vi "Process.vi"(0 "reference in":refnum<class "Active object Event.lvclass">, 5 "error in (no error)":errorcluster) -> (14 "reference out":refnum<class "Active object Event.lvclass">, 19 "error out":errorcluster)   [LabVIEW 2019, in "Active object Event.lvclass"]
uses:
  Active object Event.lvclass
panel:
  out "Last Command":string
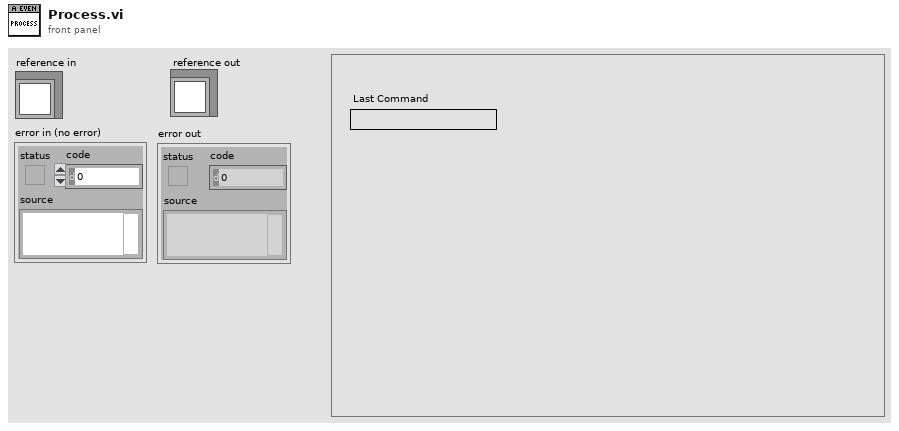
[diagram p1: front panel]
types:
  T1 = cluster{"Event":refnum<event-registration>, "Command":string, "Data":variant}
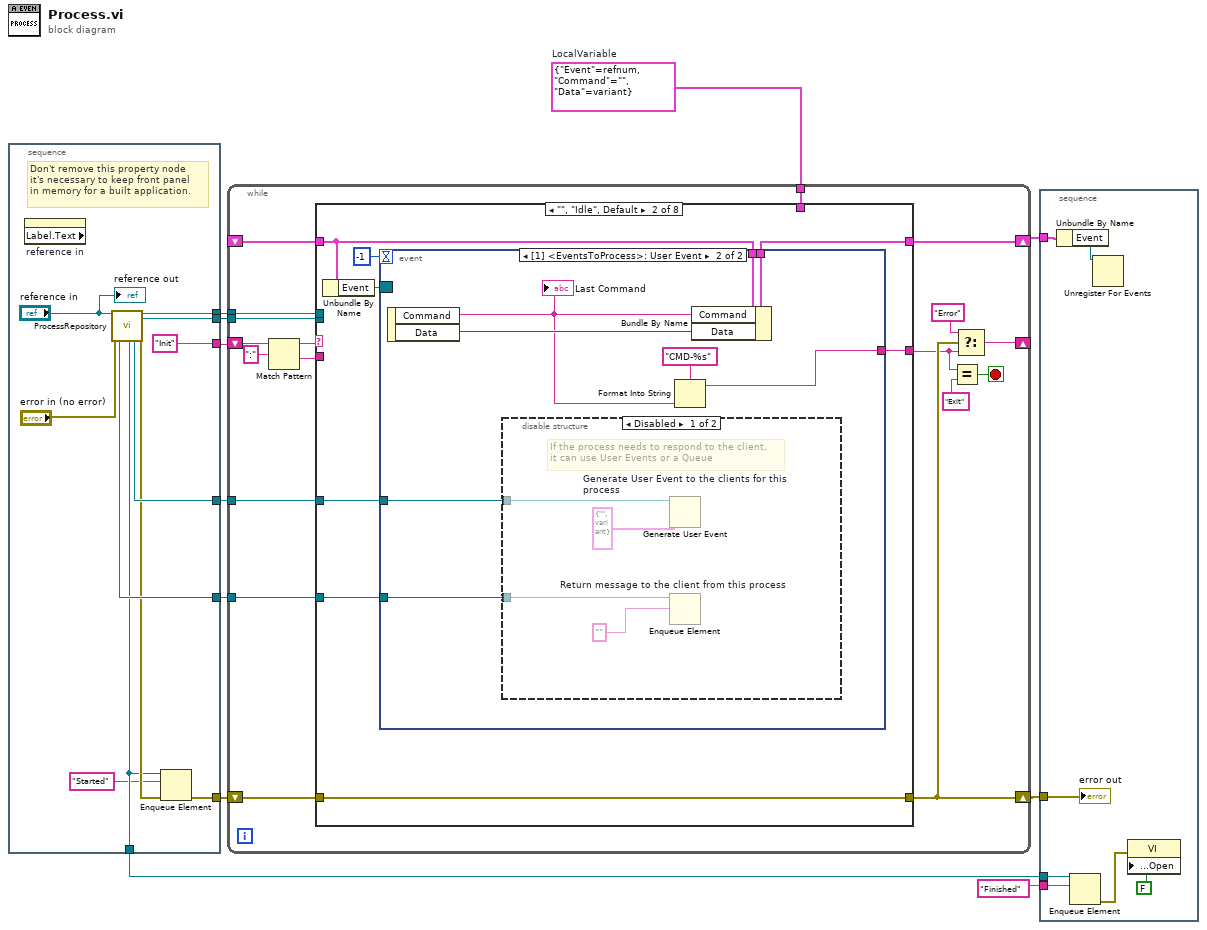
[diagram p0: block diagram]
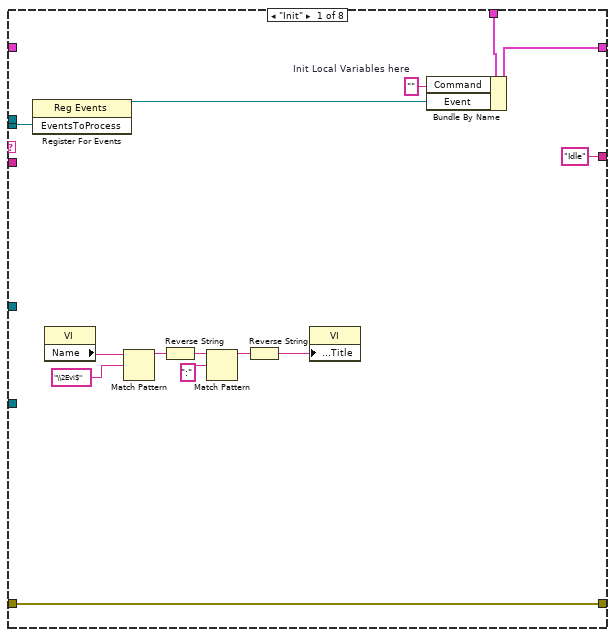
[diagram p2: hidden frame]
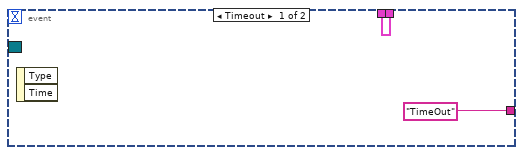
[diagram p3: hidden frame]
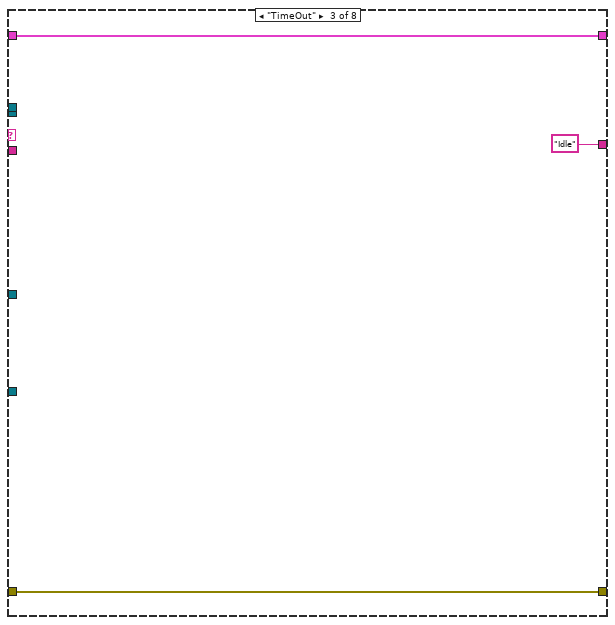
[diagram p5: hidden frame]
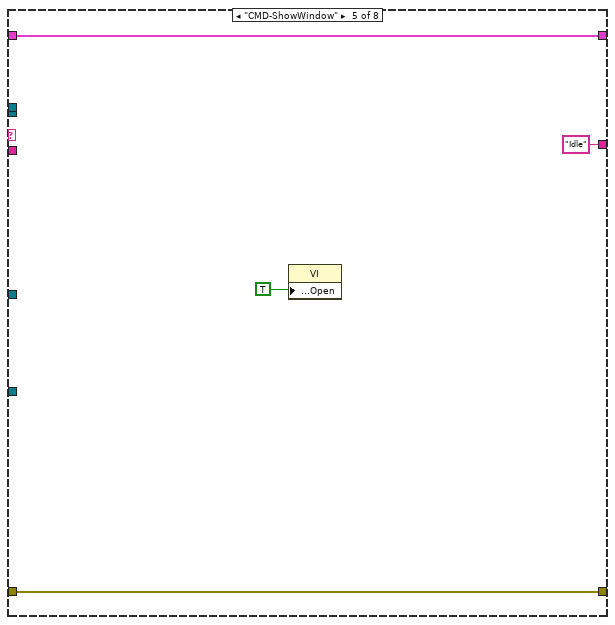
[diagram p7: hidden frame]
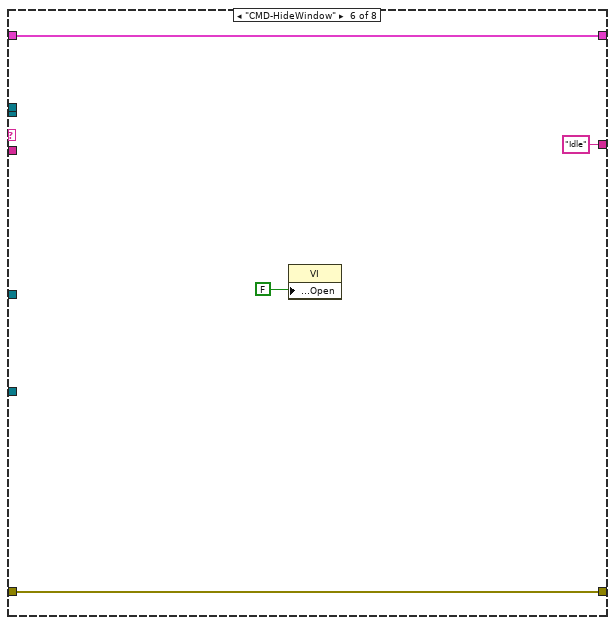
[diagram p8: hidden frame]
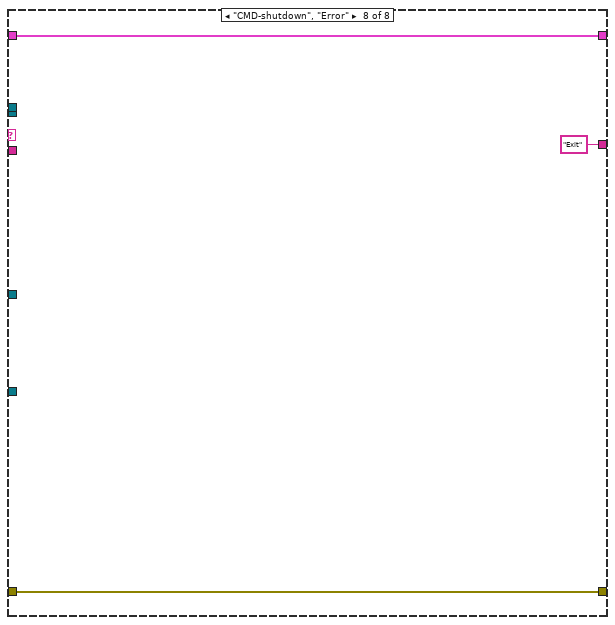
[diagram p10: hidden frame]
diagram:
  w5 = T1 {"Event"=refnum, "Command"="", "Data"=variant}  # LocalVariable
  n1 = stacked-sequence {
    tunnel: [w13] -> w11
    tunnel: [w22] -> w9
    tunnel: [w19] -> w8
    tunnel: [w14] -> w7
    tunnel: ["Init"] -> w6
    tunnel: [w17] -> w3
    tunnel: [w16] -> w2
    frame #0 {
      # "Don't remove this property node\nit's necessary to keep front panel\nin memory for a built application."
      n2 = property on="reference in" class="LVClassControl (strict)" props=["Label", "Text"]() -> ()  [unwired: 2 in, 3 out]
      n3 = call "ProcessRepository.vi"("reference in"="reference in", "error in (no error)"="error in (no error)") -> ("QueueFromProcess"=w16:refnum<queue>, "ProcessSyncQueue"=w14:refnum<queue>, "EventFromProcess"=w17:refnum<user-event>, "reference out"=w22:refnum<class "Active object Event.lvclass">, "EventsToProcess"=w19:refnum<user-event>, "error out"=w15:errorcluster)  [unwired: 10 in, 2 out]
      n4 = Enqueue Element(queue=w14, element="Started", error in (no error)=w15) -> (error out=w13:errorcluster)  [unwired: 1 in, 2 out]
      "reference out" <- "reference in"
    }
  }
  n5 = while {
    shift-right: [w33] -> w10
    shift-left: w11 -> [w38]
    tunnel: w9 -> [w39]
    tunnel: w8 -> [w40]
    shift-right: [w31] -> _
    shift-left: w6 -> [w36]
    shift-right: [w27] -> w4
    shift-left: _ -> [w26]
    tunnel: w5 -> [w25]
    tunnel: w3 -> [w24]
    tunnel: w2 -> [w23]
    stop <- w28 stop-if-true
    n6 = Match Pattern(string=w36, regular expression=":") -> (before substring=w35:string, after substring=w34:string)  [unwired: 1 in, 2 out]
    n7 = case shown="\"\", \"Idle\", Default" w35 {
      tunnel: w38 -> [w52 w57 w79 w81 w85 w89 w91 w94]
      tunnel: [w52 w57 w79 w81 w85 w89 w91 w94] -> w33
      tunnel: w40 -> [w50 _ _ _ _ _ _ _]
      tunnel: w39 -> [_ _ _ _ _ _ _ _]
      tunnel: w34 -> [_ _ _ _ _ _ _ _]
      tunnel: ["Idle" ("t") w62 "Idle" ("t") _ "Idle" ("t") "Idle" ("t") _ "Exit" ("y")] -> w30
      tunnel: [w54 w61 w77 w80 w84 w88 w90 w92] -> w27
      tunnel: w26 -> [_ w60 w77 w80 w84 w88 w90 w92]
      tunnel: w25 -> [w48 _ _ _ _ _ _ _]
      tunnel: w24 -> [_ w56 _ _ _ _ _ _]
      tunnel: w23 -> [_ w55 _ _ _ _ _ _]
      frame "Init" {
        w53 = ""  # Init Local Variables here
        n8 = register-events(w50) -> (reference out=w49:refnum<event-registration>)  [unwired: 2 in, 1 out]
        n9 = property class="VI"() -> ("Name"=w47:string)  [unwired: 2 in, 2 out]
        n10 = Match Pattern(string=w47, regular expression="\\2Evi$") -> (before substring=w45:string)  [unwired: 1 in, 3 out]
        n11 = Reverse String(1:w45) -> (0:w44:string)
        n12 = Match Pattern(string=w44, regular expression=":") -> (before substring=w42:string)  [unwired: 1 in, 3 out]
        n13 = Reverse String(1:w42) -> (0:w41:string)
        n14 = property class="VI"("Front Panel.Title"=w41) -> ()  [unwired: 2 in, 2 out]
        n15 = Bundle By Name(cluster=w48, "Command"=w53, "Event"=w49) -> (w54:T1)
      }
      frame "", "Idle", Default {
        n16 = Unbundle By Name(w60) -> ("Event"=w59:refnum<event-registration>)
        n17 = event shown="[1] <EventsToProcess>: User Event" {
          selector: w59 -> [_ _]
          dyn-events: _ -> [_ _]
          timeout: -1 -> [_ _]
          tunnel: ["TimeOut" ("t") w68] -> w62
          tunnel: w60 -> [w63 w72]
          tunnel: [w63 w71] -> w61
          tunnel: w56 -> [_ w66]
          tunnel: w55 -> [_ w65]
          event Timeout {
            n18 = event-data() -> ()  [unwired: 1 in, 2 out]
          }
          event User Event {
            n19 = event-data() -> ("Command"=w67:string, "Data"=w70:variant)  [unwired: 1 in]
            "Last Command" <- w67
            n20 = disable-structure shown="Disabled" {
              disable-tunnel: w66 -> [w76 _]
              disable-tunnel: w65 -> [w75 _]
              frame Disabled {
                # "If the process needs to respond to the client,\nit can use User Events or a Queue"
                n21 = Generate User Event "Generate User Event to the clients for this process"(user event=w76, event data cluster=cluster{"Command":string, "Data":variant} {"Command"="", "Data"=variant} ("event data")) -> ()  [unwired: 2 in, 2 out]
                n22 = Enqueue Element "Return message to the client from this process"(queue=w75, element="") -> ()  [unwired: 2 in, 3 out]
              }
              frame Enabled {
              }
            }
            n23 = Format Into String(format string="CMD-%s", w67) -> (resulting string=w68:string)  [unwired: 2 in, 1 out]
            n24 = Bundle By Name(cluster=w72, "Command"=w67, "Data"=w70) -> (w71:T1)
          }
        }
      }
      frame "TimeOut" {
      }
      frame "---- COMMANDS START----" {
      }
      frame "CMD-ShowWindow" {
        n25 = property class="VI"("Front Panel.Open"=TRUE ("Front Panel Window:Open")) -> ()  [unwired: 2 in, 2 out]
      }
      frame "CMD-HideWindow" {
        n26 = property class="VI"("Front Panel.Open"=FALSE ("Front Panel Window:Open")) -> ()  [unwired: 2 in, 2 out]
      }
      frame "----- COMMANDS END ----" {
      }
      frame "CMD-shutdown", "Error" {
      }
    }
    n27 = Equal?(x=w30, y="Exit") -> (x = y?=w28:bool)
    n28 = Select(t="Error", s=w33, f=w30) -> (s? t:f=w31:string)
  }
  n29 = stacked-sequence {
    tunnel: w10 -> [w101]
    tunnel: w7 -> [w97]
    tunnel: w4 -> [w100]
    tunnel: "Finished" ("element") -> [w95]
    frame #0 {
      n30 = Unbundle By Name(w100) -> ("Event"=w99:refnum<event-registration>)
      n31 = Enqueue Element(queue=w97, element=w95) -> (error out=w96:errorcluster)  [unwired: 2 in, 2 out]
      n32 = Unregister For Events(event registration refnum=w99) -> ()  [unwired: 1 in, 1 out]
      n33 = property class="VI"(error in=w96, "Front Panel.Open"=FALSE ("Front Panel Window:Open")) -> ()  [unwired: 1 in, 2 out]
      "error out" <- w101
    }
  }
